vi "OSICS_Get_Wavelength_Limits_TLS-AGs.vi"(7 "OSICS slot":i32=1 min=1 max=8 step=1, 8 "error in":errorcluster, 10 "nm/Freq":bool, 11 "VISA IN":refnum<visa-resource-name>) -> (0 "error out":errorcluster, 1 "WL Max/Freq Min":dbl format="%.3f", 2 "WL Min/Freq Max":dbl format="%.3f", 3 "VISA OUT":refnum<visa-resource-name>, 5 "ERR":i32)   [LabVIEW 2014, in "OSICS_LIB.lvlib"]
doc: "This Vi reads the wavelength limits of OSICS module TLS-AG depending on the input Wavelength/Frequency unit."
uses:
  OSICS_LIB.lvlib
panel:
  # "Basic Function to read the wavelength limits \nof the OSICS' TLS-AG modules"
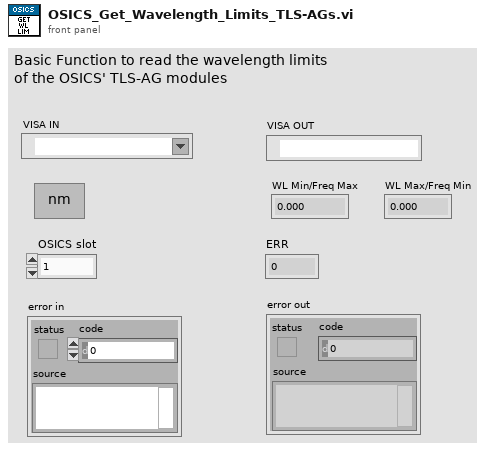
[diagram p1: front panel]
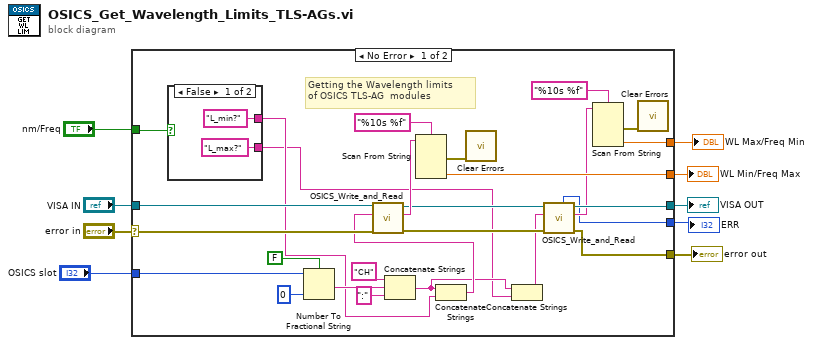
[diagram p0: block diagram]
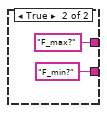
[diagram p2: hidden frame]
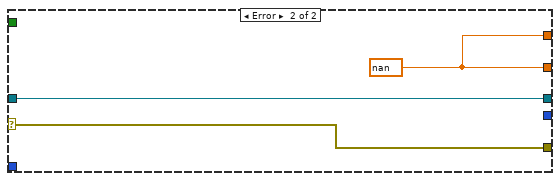
[diagram p3: hidden frame]
diagram:
  n1 = case shown="No Error" "error in" {
    selector: "error in" -> [w35 w42]
    tunnel: "VISA IN" -> [w36 w43]
    tunnel: [w30 w43] -> w8
    tunnel: [w31 w42] -> w7
    tunnel: [w33 w41] -> w5
    tunnel: [w25 w41] -> w4
    tunnel: "OSICS slot" -> [w22 _]
    tunnel: [w10 _] -> w2
    tunnel: "nm/Freq" -> [w13 _]
    frame No Error {
      # "Getting the Wavelength limits\nof OSICS TLS-AG  modules"
      n2 = case shown="False" w13 {
        tunnel: ["L_min?" "F_max?"] -> w12
        tunnel: ["L_max?" "F_min?"] -> w11
        frame False {
        }
        frame True {
        }
      }
      n3 = Number To Fractional String(use system decimal point (T)=FALSE, number=w22, precision (6)=i16 0) -> (F-format string=w18:string)  [unwired: 1 in]
      n4 = Concatenate Strings("CH" ("string"), w18, ":" ("string")) -> (w15:string)
      n5 = Concatenate Strings(w15, w12) -> (w16:string)
      n6 = call "OSICS_Write_and_Read.vi"("error in (no error)"=w35, "String to Send"=w16, "VISA IN"=w36) -> ("error out"=w32:errorcluster, "Message Available"=w29:string, "VISA OUT"=w26:refnum<visa-resource-name>)  [unwired: 5 in, 1 out]
      n7 = Scan From String(format string="%10s %f", input string=w29) -> (error out=w24:errorcluster, output 2=w33:dbl)  [unwired: 5 in, 2 out]
      n8 = call <vilib>:"Clear Errors.vi"("error in (no error)"=w24) -> ()  [unwired: 5 in, 2 out]
      n9 = Concatenate Strings(w15, w11) -> (w14:string)
      n10 = call "OSICS_Write_and_Read.vi"("error in (no error)"=w32, "String to Send"=w14, "VISA IN"=w26) -> ("error out"=w31:errorcluster, "Message Available"=w27:string, "VISA OUT"=w30:refnum<visa-resource-name>, "ERR"=w10:i32)  [unwired: 5 in]
      n11 = Scan From String(format string="%10s %f", input string=w27) -> (error out=w23:errorcluster, output 2=w25:dbl)  [unwired: 5 in, 2 out]
      n12 = call <vilib>:"Clear Errors.vi"("error in (no error)"=w23) -> ()  [unwired: 5 in, 2 out]
    }
    frame Error {
      w41 = nan
    }
  }
  "error out" <- w7
  "VISA OUT" <- w8
  "WL Min/Freq Max" <- w5
  "WL Max/Freq Min" <- w4
  "ERR" <- w2
